vi "Error_Log to File (Simple).vi"(7 "Error Log Filepath":path=path "d:/", 8 "error in (no error)":errorcluster, 10 "Error Data_IN":errorcluster, 11 "Error Log Filename":string) -> (0 "error out":errorcluster, 2 "Error Data_OUT":errorcluster, 3 "1D Error Array (String)":string[](array[string]))   [LabVIEW 2010]
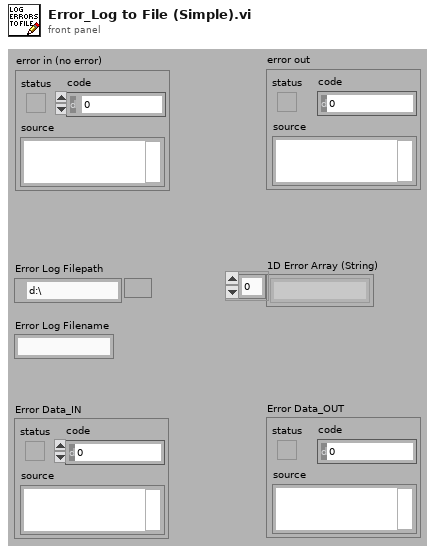
[diagram p1: front panel]
types:
  T1 = enum16{"open", "replace", "create", "open or create", "replace or create", "replace or create with confirmation"}
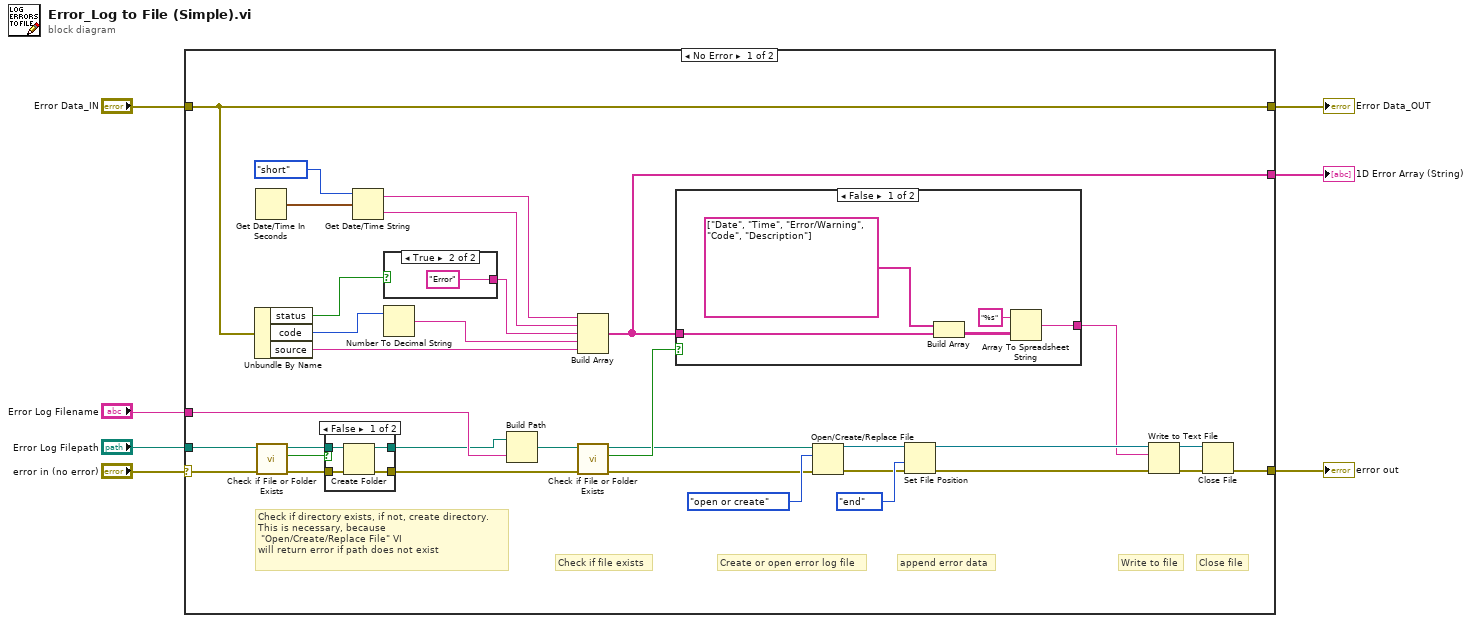
[diagram p0: block diagram]
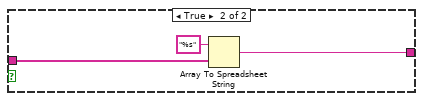
[diagram p3: hidden frame]
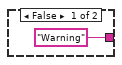
[diagram p4: hidden frame]
diagram:
  n1 = case shown="No Error" "error in (no error)" {
    selector: "error in (no error)" -> [w19 w58]
    tunnel: "Error Log Filepath" -> [w18 _]
    tunnel: [w32 w58] -> w6
    tunnel: "Error Log Filename" -> [w31 _]
    tunnel: "Error Data_IN" -> [w8 w57]
    tunnel: [w25 _] -> w2
    tunnel: [w8 w57] -> w1
    frame No Error {
      # "Close file"
      # "Write to file"
      # "Check if file exists"
      # "append error data"
      # "Check if directory exists, if not, create directory.\nThis is necessary, because\n \"Open/Create/Replace File\" VI\nwill return error if path does not exist"
      # "Create or open error log file"
      n2 = Unbundle By Name(w8) -> ("status"=w27:bool, "code"=w30:i32, "source"=w28:string)
      n3 = Get Date/Time In Seconds() -> (seconds since 1Jan1904=w12:timestamp)
      n4 = call <vilib>:"Check if File or Folder Exists.vi"("error in (no error)"=w19, "path"=w18) -> ("error out"=w17:errorcluster, "file or folder exists?"=w14:bool, "dup path"=w15:path)  [unwired: 7 in]
      n5 = case shown="False" w14 {
        tunnel: w17 -> [w44 w46]
        tunnel: [w43 w46] -> w16
        tunnel: w15 -> [w42 w45]
        tunnel: [w41 w45] -> w13
        frame False {
          n6 = Create Folder(path (use dialog)=w42, error in=w44) -> (created path=w41:path, error out=w43:errorcluster)  [unwired: 1 in, 1 out]
        }
        frame True {
        }
      }
      n7 = Get Date/Time String(date format (0)=enum16{"short", "long", "abbreviated"}."short", seconds (now)=w12) -> (date string=w11:string, time string=w10:string)  [unwired: 1 in]
      n8 = case shown="True" w27 {
        tunnel: ["Warning" "Error"] -> w26
        frame False {
        }
        frame True {
        }
      }
      n9 = Number To Decimal String(number=w30) -> (decimal integer string=w29:string)  [unwired: 1 in]
      n10 = Build Path(base path=w13, name or relative path=w31) -> (appended path=w24:path)
      n11 = Build Array(w11, w10, w26, w29, w28) -> (w25:string[])
      n12 = call <vilib>:"Check if File or Folder Exists.vi"("error in (no error)"=w16, "path"=w24) -> ("error out"=w23:errorcluster, "file or folder exists?"=w22:bool, "dup path"=w20:path)  [unwired: 7 in]
      n13 = case shown="False" w22 {
        tunnel: w25 -> [w48 w53]
        tunnel: [w50 w52] -> w21
        frame False {
          n14 = Build Array(string[] ["Date", "Time", "Error/Warning", "Code", "Description"] ("element"), w48) -> (w49:string[][])
          n15 = Array To Spreadsheet String(array=w49, 3:"%s" ("format string")) -> (spreadsheet string=w50:string)  [unwired: 1 in]
        }
        frame True {
          n16 = Array To Spreadsheet String(array=w53, 3:"%s" ("format string")) -> (spreadsheet string=w52:string)  [unwired: 1 in]
        }
      }
      n17 = Open/Create/Replace File(file path (use dialog)=w20, error in=w23, operation (0:open)=T1."open or create") -> (refnum out=w33:refnum<file>, error out=w34:errorcluster)  [unwired: 3 in, 1 out]
      n18 = Set File Position(refnum=w33, from (0:start)=enum16{"start", "end", "current"}."end", error in=w34) -> (refnum out=w38:refnum<file>, error out=w37:errorcluster)  [unwired: 1 in]
      n19 = Write to Text File(file (use dialog)=w38, text=w21, error in=w37) -> (refnum out=w40:refnum<file>, error out=w39:errorcluster)  [unwired: 1 in, 1 out]
      n20 = Close File(refnum=w40, error in=w39) -> (error out=w32:errorcluster)  [unwired: 1 out]
    }
    frame Error {
    }
  }
  "error out" <- w6
  "1D Error Array (String)" <- w2
  "Error Data_OUT" <- w1
